vi "plate_zero_v2 - 副本.vi"(8 "error in":errorcluster, 10 "DO array":bool[](array[boolean]), 11 "tasks":T1) -> (0 "error out":errorcluster)   [LabVIEW 2013]
uses:
  <vilib>/DAQmx/write.llb/DAQmx Write (Digital 1D Bool NChan 1Samp 1Line).vi
  <vilib>/DAQmx/read.llb/DAQmx Read (Digital 1D Bool NChan 1Samp 1Line).vi
  <vilib>/DAQmx/configure/timing.llb/DAQmx Timing (Implicit).vi
  <vilib>/DAQmx/miscellaneous.llb/DAQmx Fill In Error Info.vi
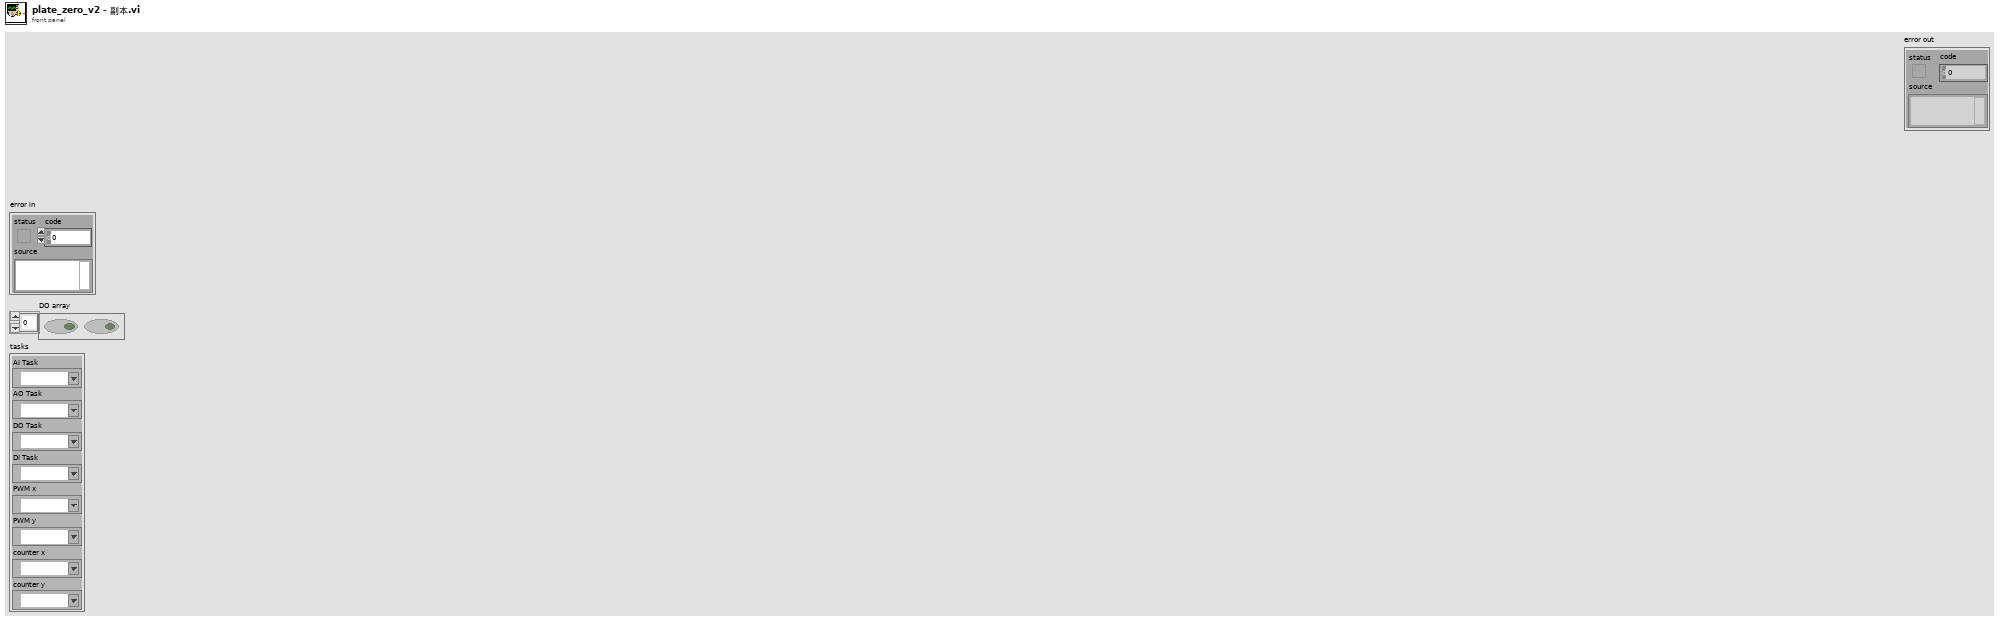
[diagram p1: front panel]
types:
  T1 = cluster{"AI Task":refnum<k21>, "AO Task":refnum<k21>, "DO Task":refnum<k21>, "DI Task":refnum<k21>, "PWM x":refnum<k21>, "PWM y":refnum<k21>, "counter x":refnum<k21>, "counter y":refnum<k21>}
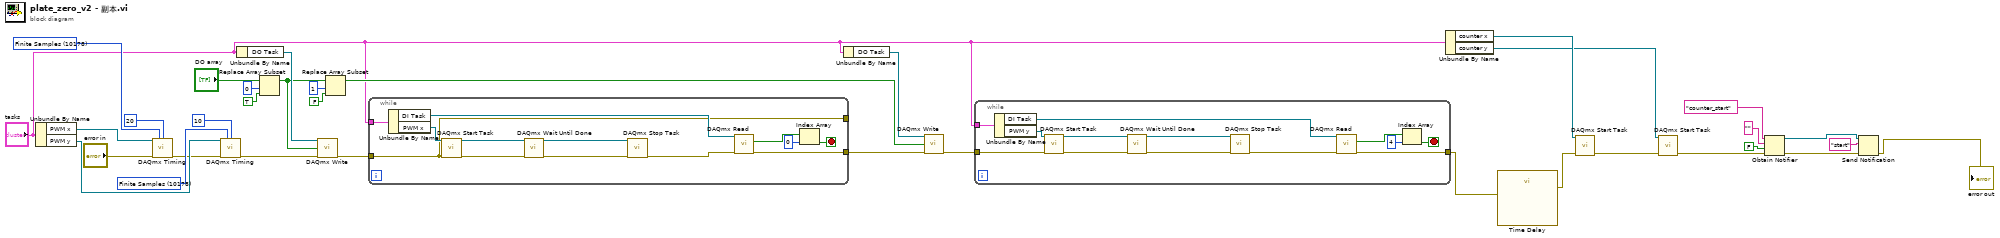
[diagram p0: block diagram]
diagram:
  w32 = 10178 items=["Finite Samples"=10178, "Continuous Samples"=10123, "Hardware Timed Single Point"=12522] ("sample mode")
  w34 = 10178 items=["Finite Samples"=10178, "Continuous Samples"=10123, "Hardware Timed Single Point"=12522] ("sample mode")
  n1 = Unbundle By Name("tasks") -> ("PWM x"=w35:refnum<k21>, "PWM y"=w30:refnum<k21>)
  n2 = call-poly <vilib>:"DAQmx Timing.vi"("task/channels in"=w35, "sample mode"=w34, "samples per channel"=20, "error in"="error in") -> ("error out"=w29:errorcluster)  [unwired: 10 in, 1 out]
  n3 = call-poly <vilib>:"DAQmx Timing.vi"("task/channels in"=w30, "sample mode"=w32, "samples per channel"=10, "error in"=w29) -> ("error out"=w17:errorcluster)  [unwired: 10 in, 1 out]
  n4 = Unbundle By Name("tasks") -> ("DO Task"=w25:refnum<k21>)
  n5 = Replace Array Subset(array="DO array", new element=TRUE ("new element/subarray"), index=0) -> (w22:bool[])
  n6 = call-poly <vilib>:"DAQmx Write.vi"("task/channels in"=w25, "data"=w22, "error in"=w17) -> ("error out"=w28:errorcluster)  [unwired: 10 in, 2 out]
  n7 = Replace Array Subset "Replace Array Subset"(array=w22, new element=FALSE ("new element/subarray"), index=1) -> (w5:bool[])
  n8 = while {
    tunnel: [w36] -> _
    tunnel: "tasks" -> [w48]
    tunnel: [w37] -> w16
    tunnel: w28 -> [w36]
    stop <- w44 stop-if-true
    n9 = Unbundle By Name(w48) -> ("DI Task"=w47:refnum<k21>, "PWM x"=w43:refnum<k21>)
    n10 = call <vilib>:"DAQmx Start Task.vi"("task/channels in"=w43, "error in"=w36) -> ("task out"=w41:refnum<k21>, "error out"=w42:errorcluster)  [unwired: 12 in]
    n11 = call <vilib>:"DAQmx Wait Until Done.vi"("task/channels in"=w41, "error in"=w42) -> ("task out"=w38:refnum<k21>, "error out"=w40:errorcluster)  [unwired: 12 in]
    n12 = call <vilib>:"DAQmx Stop Task.vi"("task/channels in"=w38, "error in"=w40) -> ("error out"=w39:errorcluster)  [unwired: 12 in, 1 out]
    n13 = call-poly <vilib>:"DAQmx Read.vi"("task/channels in"=w47, "error in"=w39) -> ("data"=w46:bool[], "error out"=w37:errorcluster)  [unwired: 11 in, 1 out]
    n14 = Index Array(array=w46, index=0) -> (element=w44:bool)
  }
  n15 = Unbundle By Name("tasks") -> ("DO Task"=w23:refnum<k21>)
  n16 = call-poly <vilib>:"DAQmx Write.vi"("task/channels in"=w23, "data"=w5, "error in"=w16) -> ("error out"=w24:errorcluster)  [unwired: 10 in, 2 out]
  n17 = while {
    tunnel: "tasks" -> [w61]
    tunnel: [w50] -> w2
    tunnel: w24 -> [w49]
    stop <- w57 stop-if-true
    n18 = Unbundle By Name(w61) -> ("DI Task"=w60:refnum<k21>, "PWM y"=w56:refnum<k21>)
    n19 = call <vilib>:"DAQmx Start Task.vi"("task/channels in"=w56, "error in"=w49) -> ("task out"=w54:refnum<k21>, "error out"=w55:errorcluster)  [unwired: 12 in]
    n20 = call <vilib>:"DAQmx Wait Until Done.vi"("task/channels in"=w54, "error in"=w55) -> ("task out"=w51:refnum<k21>, "error out"=w53:errorcluster)  [unwired: 12 in]
    n21 = call <vilib>:"DAQmx Stop Task.vi"("task/channels in"=w51, "error in"=w53) -> ("error out"=w52:errorcluster)  [unwired: 12 in, 1 out]
    n22 = call-poly <vilib>:"DAQmx Read.vi"("task/channels in"=w60, "error in"=w52) -> ("data"=w59:bool[], "error out"=w50:errorcluster)  [unwired: 11 in, 1 out]
    n23 = Index Array(array=w59, index=4) -> (element=w57:bool)
  }
  n24 = Unbundle By Name("tasks") -> ("counter x"=w12:refnum<k21>, "counter y"=w11:refnum<k21>)
  n25 = call "Time Delay"("error in (no error)"=w2) -> ("error out"=w1:errorcluster)  [unwired: 10 in]
  n26 = call <vilib>:"DAQmx Start Task.vi"("task/channels in"=w12, "error in"=w1) -> ("error out"=w10:errorcluster)  [unwired: 12 in, 1 out]
  n27 = call <vilib>:"DAQmx Start Task.vi"("task/channels in"=w11, "error in"=w10) -> ("error out"=w9:errorcluster)  [unwired: 12 in, 1 out]
  n28 = Obtain Notifier(name (unnamed)="counter_start", notification data type="", create if not found? (T)=FALSE, error in (no error)=w9) -> (notifier out=w7:refnum<notifier>, error out=w8:errorcluster)  [unwired: 1 out]
  n29 = Send Notification(notification="start", notifier=w7, error in (no error)=w8) -> (error out=→"error out":errorcluster)  [unwired: 1 out]
